vi "initial_function.vi"   [LabVIEW 2016]
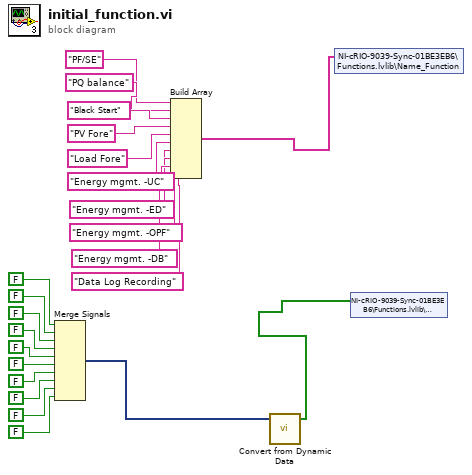
[diagram p0: block diagram]
diagram:
  n1 = Merge Signals(FALSE ("State3"), FALSE ("State3"), FALSE ("State3"), FALSE ("State3"), FALSE ("State3"), FALSE ("State3"), FALSE ("State3"), FALSE ("State3"), FALSE ("State3"), FALSE ("State3")) -> (w13:dynamicdata)
  n2 = Build Array("PF/SE", "PQ balance", "Black Start", "PV Fore", "Load Fore", "Energy mgmt. -UC", "Energy mgmt. -ED", "Energy mgmt. -OPF", "Energy mgmt. -DB", "Data Log Recording") -> (w2:string[])
  n3 = call "Convert from Dynamic Data"("Dynamic Data Type"=w13) -> ("Array"=w1:bool[])  [unwired: 3 in]
  n4 = shared-variable "NI-cRIO-9039-Sync-01BE3EB6\\Functions.lvlib\\Name_Function"(w2) -> ()  [unwired: 1 in, 1 out]
  n5 = shared-variable "NI-cRIO-9039-Sync-01BE3EB6\\Functions.lvlib\\Functions"(w1) -> ()  [unwired: 1 in, 1 out]
